vi "fix_ICS_msg.vi"(11 "Msg in":string) -> (3 "JSON":string)   [LabVIEW 2018]
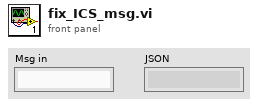
[diagram p1: front panel]
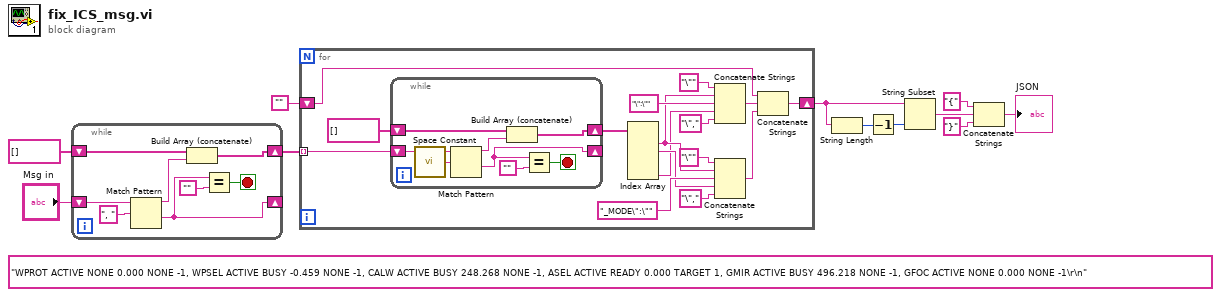
[diagram p0: block diagram]
diagram:
  (unwired) "WPROT ACTIVE NONE 0.000 NONE -1, WPSEL ACTIVE BUSY -0.459 NONE -1, CALW ACTIVE BUSY 248.268 NONE -1, ASEL ACTIVE READY 0.000 TARGET 1, GMIR ACTIVE BUSY 496.218 NONE -1, GFOC ACTIVE NONE 0.000 NONE -1\r\n" ("search string/char (-)")
  n1 = while {
    shift-right: [w16] -> w2
    shift-left: string[] [] -> [w17]
    shift-right: [w12] -> _
    shift-left: "Msg in" -> [w15]
    stop <- w18 stop-if-true
    n2 = Match Pattern(string=w15, regular expression=", " ("search string/char (-)")) -> (before substring=w13:string, after substring=w12:string)  [unwired: 1 in, 2 out]
    n3 = Build Array (concatenate)(w17, w13) -> (w16:string[])
    n4 = Equal?(x=w12, y="") -> (x = y?=w18:bool)
  }
  n5 = for {
    tunnel: w2 -> [w34] mode=indexing
    shift-right: [w22] -> w4
    shift-left: "" -> [w21]
    n6 = while {
      shift-right: [w40] -> w33
      shift-left: string[] [] -> [w41]
      shift-right: [w37] -> _
      shift-left: w34 -> [w39]
      stop <- w42 stop-if-true
      n7 = call <vilib>:"Space Constant.vi"() -> ("String"=w36:string)
      n8 = Match Pattern(string=w39, regular expression=w36) -> (before substring=w38:string, after substring=w37:string)  [unwired: 1 in, 2 out]
      n9 = Build Array (concatenate)(w41, w38) -> (w40:string[])
      n10 = Equal?(x=w37, y="") -> (x = y?=w42:bool)
    }
    n11 = Index Array(array=w33) -> (element #1=w26:string, element #2=w25:string, element #5=w20:string)  [unwired: 5 in, 2 out]
    n12 = Concatenate Strings("\"" ("search string/char (-)"), w26, "\":\"" ("search string/char (-)"), w20, "\"," ("search string/char (-)")) -> (w23:string)
    n13 = Concatenate Strings("\"" ("search string/char (-)"), w26, "_MODE\":\"" ("search string/char (-)"), w25, "\"," ("search string/char (-)")) -> (w24:string)
    n14 = Concatenate Strings(w21, w23, w24) -> (w22:string)
  }
  n15 = String Length(string=w4) -> (length=w6:i32)
  n16 = Decrement(x=w6) -> (x-1=w5:i32)
  n17 = String Subset(string=w4, length (rest)=w5) -> (substring=w7:string)  [unwired: 1 in]
  n18 = Concatenate Strings("{" ("search string/char (-)"), w7, "}" ("search string/char (-)")) -> (→"JSON":string)
